vi "StopFGV.vi"(8 "error in":errorcluster, 10 "STOP":bool, 11 "Enum":enum16{"init", "write", "read"}(ring)) -> (0 "error out":errorcluster, 3 "STOP Out":bool)   [LabVIEW 2026]
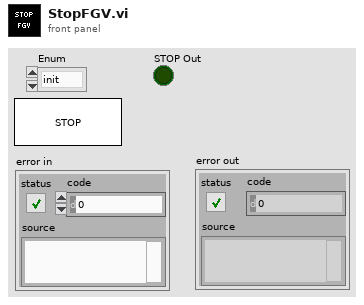
[diagram p1: front panel]
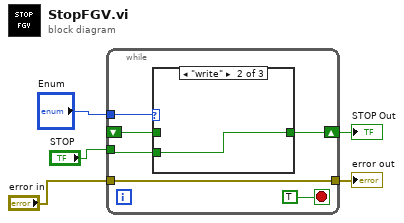
[diagram p0: block diagram]
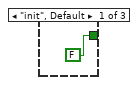
[diagram p2: hidden frame]
diagram:
  n1 = while {
    tunnel: "Enum" -> [w11]
    tunnel: "STOP" -> [w8]
    shift-right: [w9] -> w3
    shift-left: _ -> [w7]
    tunnel: "error in" -> [w6]
    tunnel: [w6] -> w1
    stop <- TRUE stop-if-true
    n2 = case shown="\"write\"" w11 {
      tunnel: [FALSE ("STOP") w13 w14] -> w9
      tunnel: w8 -> [_ w13 _]
      tunnel: w7 -> [_ _ w14]
      frame "init", Default {
      }
      frame "write" {
      }
      frame "read" {
      }
    }
  }
  "STOP Out" <- w3
  "error out" <- w1
